vi "Dynamic launcher.vi"(0 "element":string[](array[string]), 1 "Clone ?":bool, 5 "Value":variant[](array[variant]), 7 "VI Refnum":refnum<vi>, 9 "vi path":path, 11 "error in (no error)":errorcluster, 12 "Open FP":bool=TRUE, 14 "options":i32=8 format="%.0x") -> (4 "reference out":refnum<vi>, 6 "Failed":bool, 15 "error out":errorcluster)   [LabVIEW 2024, in "Launcher_DTU.lvlib"]
uses:
  Launcher_DTU.lvlib
  <vilib>/Utility/error.llb/DialogType.ctl
  Dialog Box/Poly_One_Button.vi
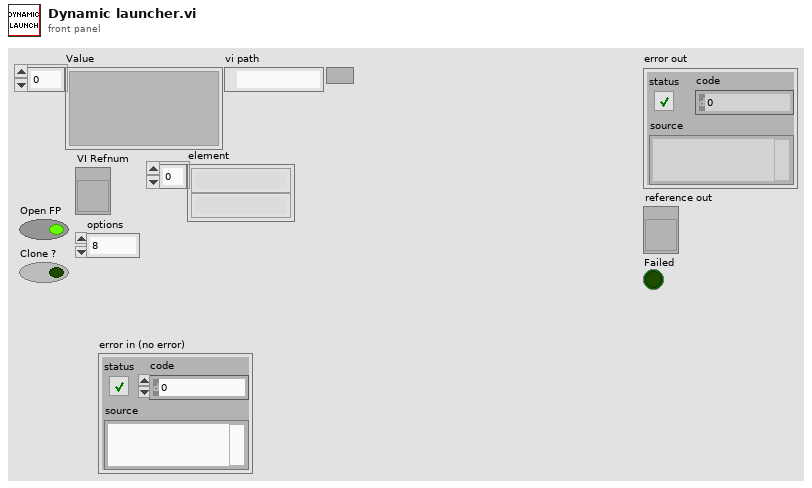
[diagram p1: front panel]
types:
  T1 = typedef "DialogType.ctl" = u16
  T2 = enum32{"Bad", "Idle", "Run top level", "Running"}
  T3 = enum32{"Invalid", "Standard", "Closed", "Hidden", "Minimized", "Maximized"}
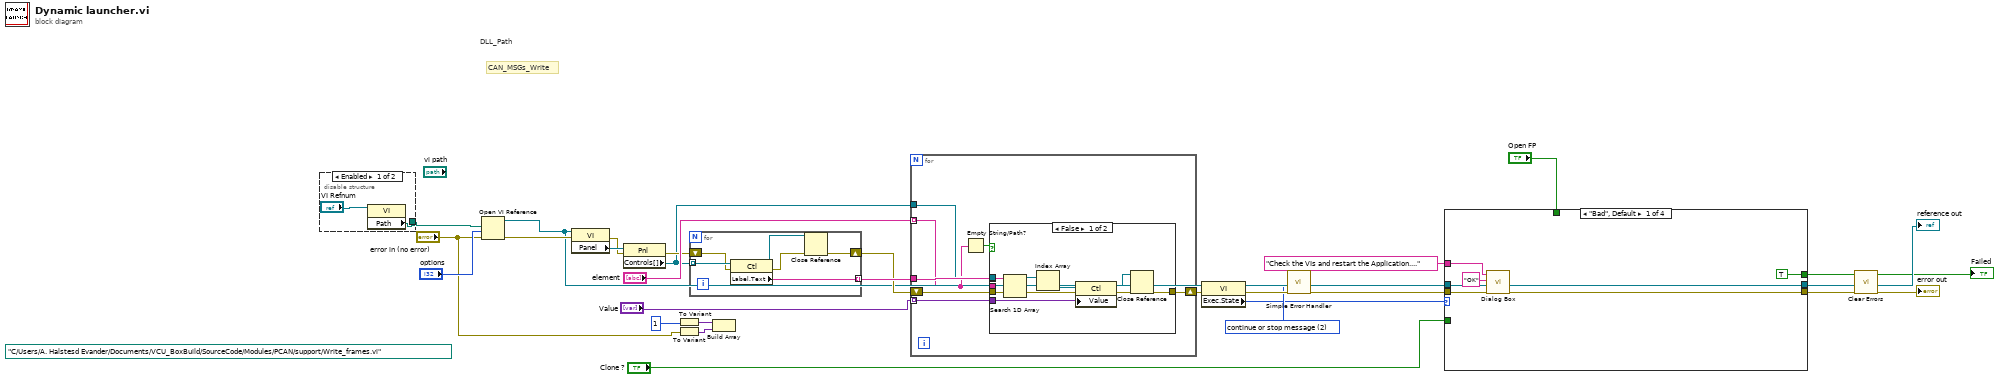
[diagram p0: block diagram]
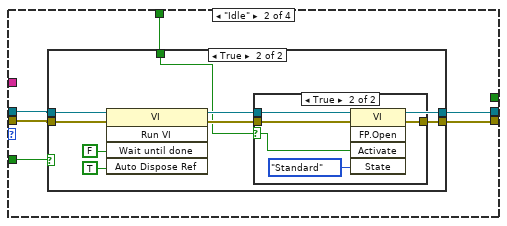
[diagram p4: hidden frame]
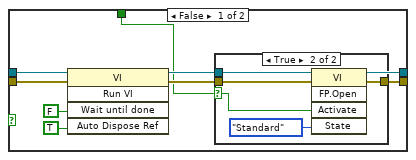
[diagram p5: hidden frame]
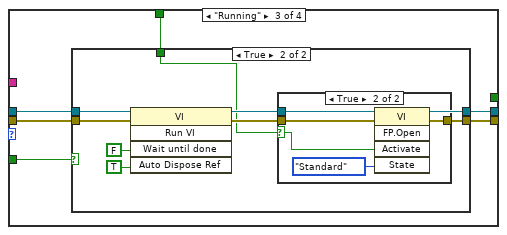
[diagram p8: hidden frame]
diagram:
  (unwired) path "C:/Users/A. Halstesd Evander/Documents/VCU_BoxBuild/SourceCode/Modules/PCAN/support/Write_frames.vi" ("VI Path")
  w12 = T1 2 items=["no dialog", "OK message", "continue or stop message", "OK message + warnings", "continue/stop + warnings"] ("type of dialog (OK msg:1)")
  # "DLL_Path"
  # "CAN_MSGs_Write"
  n1 = disable-structure shown="Enabled" {
    disable-tunnel: [w30 _] -> w1
    frame Enabled {
      n2 = property class="VI"(reference="VI Refnum") -> ("Path"=w30:path)  [unwired: 1 in, 2 out]
    }
    frame Disabled {
    }
  }
  n3 = Open VI Reference(vi path=w1, options="options", error in (no error)="error in (no error)") -> (vi reference=w8:refnum<vi>, error out=w9:errorcluster)  [unwired: 3 in]
  n4 = property class="VI"(reference=w8, error in=w9) -> (error out=w23:errorcluster, "Panel"=w24:refnum<vi>)  [unwired: 1 out]
  n5 = property class="Pnl"(reference=w24, error in=w23) -> (error out=w22:errorcluster, "Controls[]"=w20:refnum<vi>[])  [unwired: 1 out]
  n6 = To Variant(anything=1) -> (Variant=w6:variant)
  n7 = To Variant(anything="error in (no error)") -> (Variant=w5:variant)
  n8 = for {
    tunnel: w20 -> [w37] mode=indexing
    shift-right: [w33] -> w19
    shift-left: w22 -> [w36]
    tunnel: [w34] -> w21 mode=indexing
    n9 = property class="Ctl"(reference=w37, error in=w36) -> (reference out=w32:refnum<vi>, error out=w35:errorcluster, "Label.Text"=w34:string)
    n10 = Close Reference(reference=w32, error in (no error)=w35) -> (error out=w33:errorcluster)
  }
  n11 = Build Array(w6, w5) -> ()  [unwired: 1 out]
  n12 = for {
    tunnel: w21 -> [w44]
    tunnel: "element" -> [w38] mode=indexing
    tunnel: w20 -> [w43]
    tunnel: "Value" -> [w41] mode=indexing
    shift-right: [w40] -> w18
    shift-left: w19 -> [w42]
    n13 = Empty String/Path?(string/path=w38) -> (empty?=w39:bool)
    n14 = case shown="False" w39 {
      tunnel: w44 -> [w54 _]
      tunnel: w38 -> [w53 _]
      tunnel: w43 -> [w52 _]
      tunnel: w42 -> [w51 w55]
      tunnel: w41 -> [w50 _]
      tunnel: [w46 w55] -> w40
      frame False {
        n15 = Search 1D Array(1D array=w54, element=w53) -> (index of element=w49:i32)  [unwired: 1 in]
        n16 = Index Array(array=w52, index=w49) -> (element=w48:refnum<vi>)
        n17 = property class="Ctl"(reference=w48, error in=w51, "Value"=w50) -> (reference out=w45:refnum<vi>, error out=w47:errorcluster)
        n18 = Close Reference(reference=w45, error in (no error)=w47) -> (error out=w46:errorcluster)
      }
      frame True {
      }
    }
  }
  n19 = property class="VI"(reference=w8, error in=w18) -> (reference out=w16:refnum<vi>, error out=w17:errorcluster, "Exec.State"=w11:T2)
  n20 = call <vilib>:"Simple Error Handler.vi"("type of dialog (OK msg:1)"=w12, "error in (no error)"=w17) -> ("error out"=w13:errorcluster)  [unwired: 3 in, 4 out]
  n21 = case shown="\"Bad\", Default" w11 {
    tunnel: [w59 w63 w99 w118] -> w28
    tunnel: [w61 w62 w98 w119] -> w27
    tunnel: w13 -> [w60 w67 w101 w118]
    tunnel: w16 -> [w61 w66 w100 w119]
    tunnel: "Check the VIs and restart the Application...." -> [w58 _ _ _]
    tunnel: [TRUE _ _ _] -> w26
    tunnel: "Open FP" -> [_ w65 w97 _]
    tunnel: "Clone ?" -> [_ w64 w96 _]
    frame "Bad", Default {
      n22 = call-poly "Dialog Box.vi"("error in"=w60, "Button Text"="OK", "Message"=w58) -> ("error out"=w59:errorcluster)  [unwired: 7 in, 1 out]
    }
    frame "Idle" {
      n23 = case shown="True" w64 {
        tunnel: w67 -> [w74 w88]
        tunnel: w66 -> [w73 w87]
        tunnel: [w72 w86] -> w62
        tunnel: w65 -> [w69 w83]
        tunnel: [w68 w82] -> w63
        frame False {
          n24 = invoke class="VI" method="Run VI"(reference=w73, error in=w74, "Wait until done"=FALSE ("Wait Until Done"), "Auto Dispose Ref"=TRUE ("Auto Dispose Reference")) -> (reference out=w72:refnum<vi>, error out=w75:errorcluster)  [unwired: 1 in, 3 out]
          n25 = case shown="True" w69 {
            selector: w69 -> [_ w77]
            tunnel: w75 -> [w76 w81]
            tunnel: [w76 w80] -> w68
            tunnel: w72 -> [_ w79]
            frame False {
            }
            frame True {
              n26 = invoke class="VI" method="FP.Open"(reference=w79, error in=w81, "Activate"=w77, "State"=T3."Standard") -> (error out=w80:errorcluster)  [unwired: 1 in, 4 out]
            }
          }
        }
        frame True {
          n27 = invoke class="VI" method="Run VI"(reference=w87, error in=w88, "Wait until done"=FALSE ("Wait Until Done"), "Auto Dispose Ref"=TRUE ("Auto Dispose Reference")) -> (reference out=w86:refnum<vi>, error out=w89:errorcluster)  [unwired: 1 in, 3 out]
          n28 = case shown="True" w83 {
            selector: w83 -> [_ w91]
            tunnel: w89 -> [w90 w95]
            tunnel: [w90 w94] -> w82
            tunnel: w86 -> [_ w93]
            frame False {
            }
            frame True {
              n29 = invoke class="VI" method="FP.Open"(reference=w93, error in=w95, "Activate"=w91, "State"=T3."Standard") -> (error out=w94:errorcluster)  [unwired: 1 in, 4 out]
            }
          }
        }
      }
    }
    frame "Running" {
      n30 = case shown="True" w96 {
        tunnel: w101 -> [w103 w110]
        tunnel: w100 -> [w102 w109]
        tunnel: [w103 w108] -> w99
        tunnel: [w102 w107] -> w98
        tunnel: w97 -> [_ w104]
        frame False {
        }
        frame True {
          n31 = invoke class="VI" method="Run VI"(reference=w109, error in=w110, "Wait until done"=FALSE ("Wait Until Done"), "Auto Dispose Ref"=TRUE ("Auto Dispose Reference")) -> (reference out=w107:refnum<vi>, error out=w111:errorcluster)  [unwired: 1 in, 3 out]
          n32 = case shown="True" w104 {
            selector: w104 -> [_ w113]
            tunnel: w111 -> [w112 w117]
            tunnel: [w112 w116] -> w108
            tunnel: w107 -> [_ w115]
            frame False {
            }
            frame True {
              n33 = invoke class="VI" method="FP.Open"(reference=w115, error in=w117, "Activate"=w113, "State"=T3."Standard") -> (error out=w116:errorcluster)  [unwired: 1 in, 4 out]
            }
          }
        }
      }
    }
    frame "Run top level" {
    }
  }
  "reference out" <- w27
  "Failed" <- w26
  n34 = call <vilib>:"Clear Errors.vi"("error in (no error)"=w28) -> ("error out"=→"error out":errorcluster)  [unwired: 5 in, 1 out]
